vi "Inner Subtest.vi"(8 "error in (no error)":errorcluster) -> (0 "error out":errorcluster)   [LabVIEW 2013]
uses:
  classes/Test/Test.lvclass
  classes/Assert/Assert.lvclass
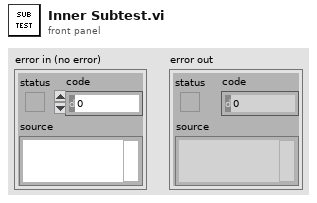
[diagram p1: front panel]
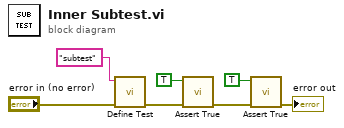
[diagram p0: block diagram]
diagram:
  n1 = call "Define Test.vi"("error in (no error)"="error in (no error)", "Label (VI Title)"="subtest") -> ("error out"=w6:errorcluster)  [unwired: 9 in]
  n2 = call "Assert True.vi"("error in (no error)"=w6, "True?"=TRUE) -> ("error out"=w1:errorcluster)  [unwired: 9 in]
  n3 = call "Assert True.vi"("error in (no error)"=w1, "True?"=TRUE) -> ("error out"=→"error out":errorcluster)  [unwired: 9 in]
